vi "Start Discovery.vi"(8 "error in (no error)":errorcluster, 11 "Vecto in":refnum<class "Vecto.lvclass">) -> (0 "error out":errorcluster, 3 "Vecto out":refnum<class "Vecto.lvclass">)   [LabVIEW 2020, in "Vecto.lvlib" / "Vecto.lvclass"]
uses:
  Vecto.lvclass
  Vecto.lvclass/Vecto.ctl
  DiscoveryService/DiscoveryService.lvclass
  Node Config/Node Config.lvclass
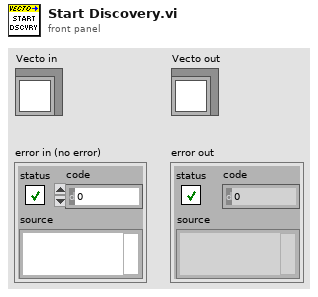
[diagram p1: front panel]
types:
  T1 = typedef "VectoConfig.lvlib/Comms Features.ctl" = cluster{"HTTP Server":bool, "TCP Messaging":bool, "Remote Data":bool, "Discovery":bool}
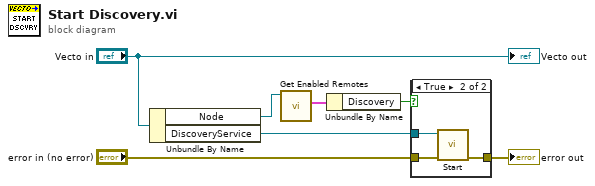
[diagram p0: block diagram]
diagram:
  n1 = Unbundle By Name("Vecto in") -> ("Node"=w3:refnum<class "Node Config.lvclass">, "DiscoveryService"=w4:refnum<class "DiscoveryService.lvclass">)
  n2 = call "Get Enabled Remotes.vi"("Node Config in"=w3) -> ("Comms Features"=w2:T1)  [unwired: 8 in, 2 out]
  n3 = Unbundle By Name(w2) -> ("Discovery"=w1:bool)
  n4 = case shown="True" w1 {
    tunnel: "error in (no error)" -> [w8 w11]
    tunnel: [w8 w10] -> w6
    tunnel: w4 -> [_ w9]
    frame False {
    }
    frame True {
      n5 = call "Start.vi"("error in (no error)"=w11, "DiscoveryService in"=w9) -> ("error out"=w10:errorcluster)  [unwired: 8 in, 1 out]
    }
  }
  "error out" <- w6
  "Vecto out" <- "Vecto in"
